vi "getKeyFormatAndValChkRes_.vi"(8 "error in":errorcluster, 9 "keyVal":string, 10 "sec":string, 11 "Tree Refnum in":refnum<vi>) -> (0 "error out":errorcluster, 1 "chkRes":string="√", 2 "keyFormat":string, 3 "Tree Refnum out":refnum<vi>)   [LabVIEW 2010]
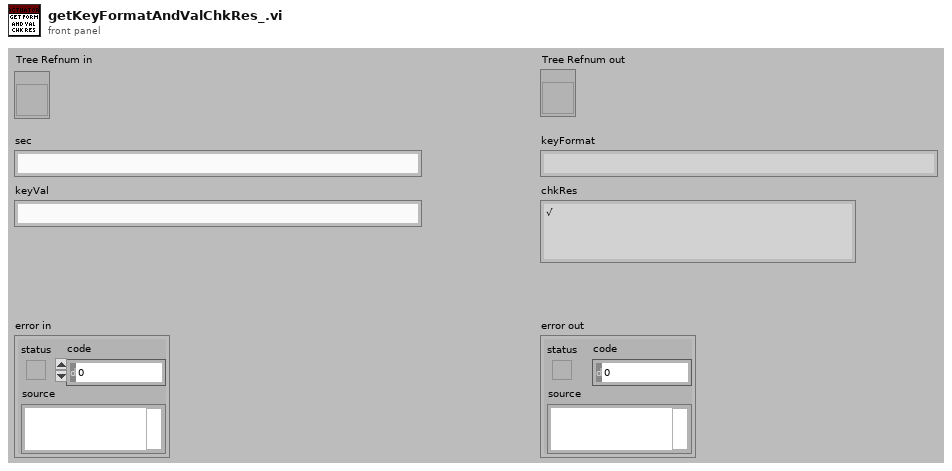
[diagram p1: front panel]
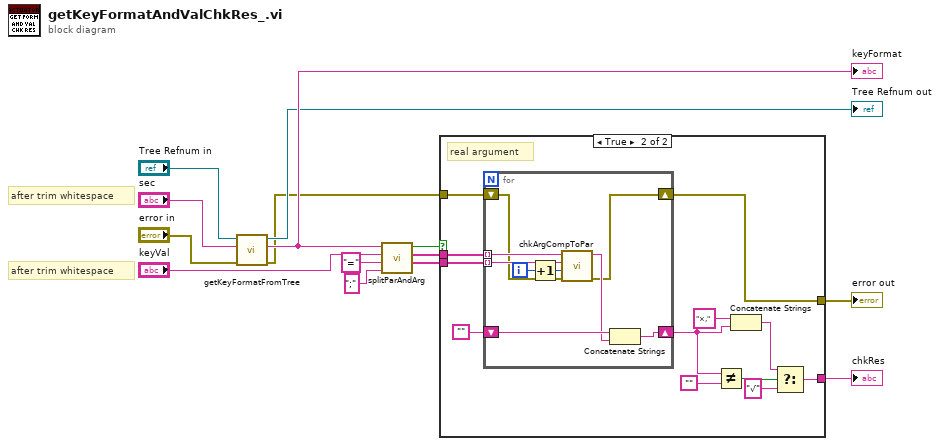
[diagram p0: block diagram]
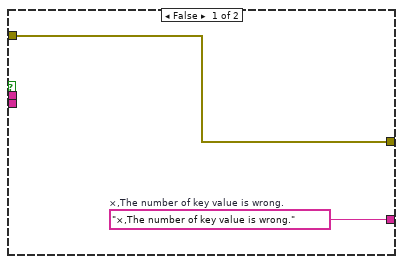
[diagram p2: hidden frame]
diagram:
  # "after trim whitespace"
  # "after trim whitespace"
  n1 = call "getKeyFormatFromTree.vi"("error in"="error in", "sec"="sec", "Tree Refnum in"="Tree Refnum in") -> ("error out"=w1:errorcluster, "keyFormat"=w6:string, "Tree Refnum out"=→"Tree Refnum out":refnum<vi>)  [unwired: 6 in]
  "keyFormat" <- w6
  n2 = call "splitParAndArg.vi"("paraEndMark"=";" ("regular expression"), "paraStartMark"="=" ("regular expression"), "allArguments"="keyVal", "allParameters"=w6) -> ("argArray"=w9:string[], "paraArray"=w8:string[], "sameNum?"=w7:bool)  [unwired: 5 in]
  n3 = case shown="True" w7 {
    tunnel: w8 -> [_ w28]
    tunnel: w9 -> [_ w27]
    tunnel: [w16 w22] -> w14
    tunnel: w1 -> [w15 w21]
    tunnel: [w15 w20] -> w13
    frame False {
      w16 = "×,The number of key value is wrong."  # ×,The number of key value is wrong.
    }
    frame True {
      # "real argument"
      n4 = for {
        tunnel: w28 -> [w37] mode=indexing
        tunnel: w27 -> [w36] mode=indexing
        shift-right: [w29] -> w18
        shift-left: "" -> [w32]
        shift-right: [w30] -> w20
        shift-left: w21 -> [w33]
        i -> [w35]
        n5 = Increment(x=w35) -> (x+1=w34:i32)
        n6 = call "chkArgCompToPar.vi"("error in"=w33, "argSN"=w34, "arg"=w36, "par"=w37) -> ("error out"=w30:errorcluster, "judgement"=w31:string)  [unwired: 6 in]
        n7 = Concatenate Strings(w32, w31) -> (w29:string)
      }
      n8 = Not Equal?(x=w18, y="") -> (x != y?=w24:bool)
      n9 = Concatenate Strings("×,", w18) -> (w17:string)
      n10 = Select(t=w17, s=w24, f="√") -> (s? t:f=w22:string)
    }
  }
  "chkRes" <- w14
  "error out" <- w13
